vi "velocitymode_rev3_ab.vi"() -> ()   [LabVIEW 2018]
uses:
  <vilib>/rvi/interface/nirviOpenFPGA/nirviOpenFPGA.xnode
  FPGA Bitfiles/WattBalanceRev1_FPGATarget_FPGASPI2_21rs6YSGst0.lvbitx
  <vilib>/rvi/interface/nirviCloseFPGA/nirviCloseFPGA.xnode
  <vilib>/FPGAPlugInAG/Dynamic/niLvFpga_Close_Dynamic.vi
  <vilib>/FPGAPlugInAG/myRIO-1900/niLvFpga_Open_myRIO-1900.vi
  <vilib>/rvi/interface/common/dynamic/niFpgaDynamicAddResources.vi
  <vilib>/Platform/TimedLoop/XDataNode/XDataNode.xnode
  <vilib>/Platform/TimedLoop/XDataNode/nitl_modes.ctl
  <vilib>/Platform/TimedLoop/XDataNode/XDNodeRunTimeDep.lvlib
  <vilib>/Platform/TimedLoop/XDataNode/wakeup.ctl
  <vilib>/Platform/TimedLoop/XDataNode/timing_clust.ctl
panel:
  out "Finished Late? [i-1]":bool
  out "BL":dbl(graph)=0.00030517112470818
  out "x/y":dbl
  out "velocity":dbl(graph)=0.00030517112470818
  out "prev pos":dbl
  in  "emf on/off":bool
  in  "pos on/off":bool
  out "Smooth EMF":dbl(graph)
  out "Smooth position":dbl(graph)=0.00030517112470818
  in  "no. moving avg.":i32=5
  in  "CH1":bool[](array[boolean])=[FALSE, FALSE, TRUE, FALSE, FALSE, TRUE, FALSE, FALSE, FALSE, FALSE, FALSE, FALSE, FALSE, FALSE, FALSE, FALSE]
  in  "CH2":bool[](array[boolean])=[FALSE, FALSE, FALSE, FALSE, FALSE, TRUE, FALSE, FALSE, FALSE, FALSE, FALSE, FALSE, FALSE, FALSE, FALSE, FALSE]
  in  "Color Box 2":u32(colorbox)
  in  "Stop Button":bool
  in  "offset (mV)":dbl
  in  "amplitude (V)":dbl
  in  "frequency (Hz)":dbl
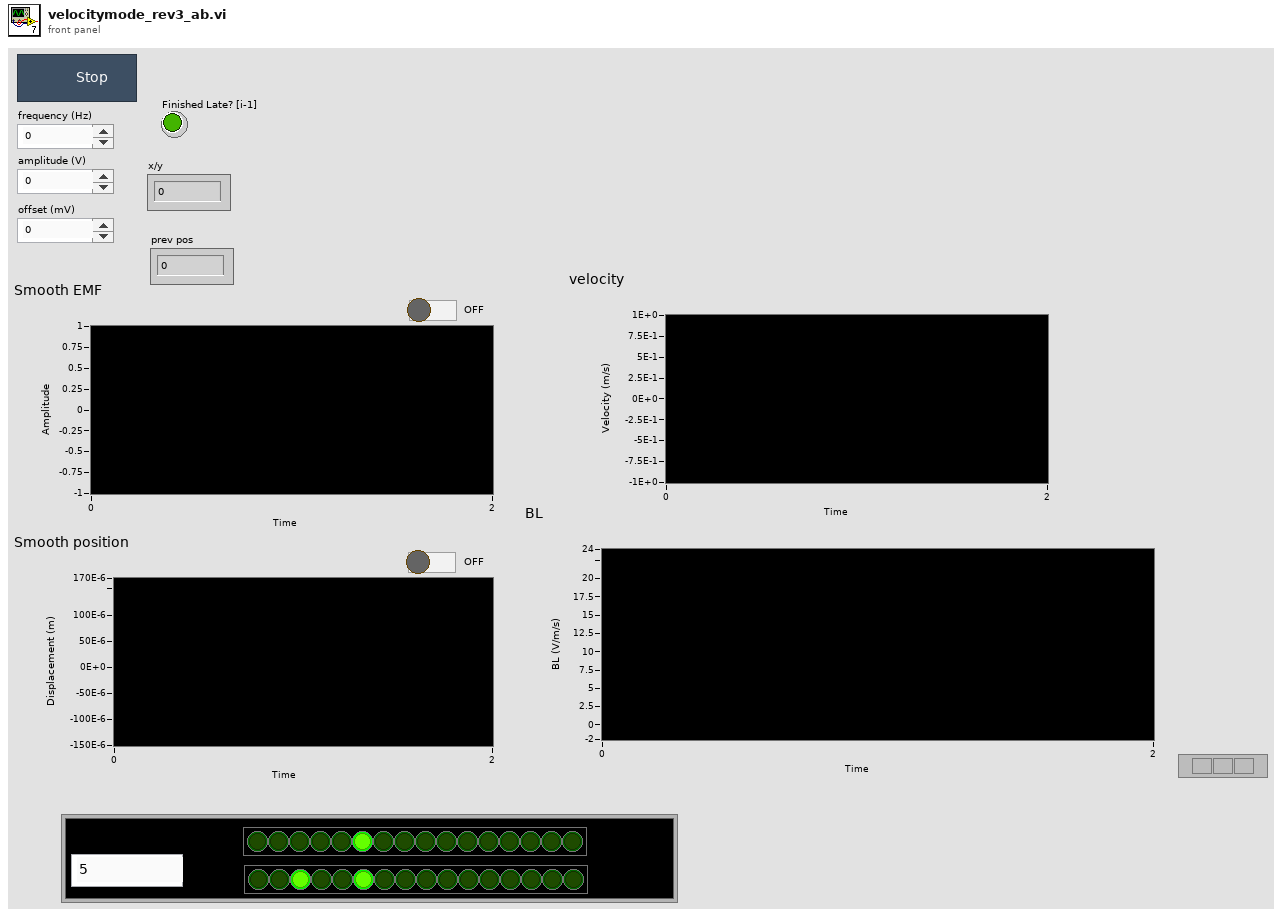
[diagram p1: front panel]
types:
  T1 = typedef "XDNodeRunTimeDep.lvlib/timing_clust.ctl" = cluster{"Expected End [f-1]":u64, "Actual End [f-1]":u64, "Finished Late? [f-1]":bool, "Expected End [i-1]":u64, "Actual End [i-1]":u64, "Finished Late? [i-1]":bool, "Expected Start [i]":u64, "Actual Start [i]":u64, "Expected Start [f]":u64, "Actual Start [f]":u64, "Source Name":string, "Structure Name":string, "Period":i64, "Deadline":i64, "Offset":i64, "Start":i64, "Priority":i32, "Timeout":i32, "Mode":T2, "Wakeup Reason":T3, "Error":errorcluster, "Source Type":string, "Secondary Source Type":string, "Global End Time":u64, "Global Start Time":u64, "Frame Duration":u64, "Iteration Duration":u64, "Assigned CPU":i32, "I/O Scan Engine Mode":u32}
  T2 = typedef "XDNodeRunTimeDep.lvlib/nitl_modes.ctl" = enum32{"No Change", "Process missed periods, maintain original phase", "Discard missed periods, maintain original phase", "Process missed periods, ignore original phase", "Discard missed periods, ignore original phase"}
  T3 = typedef "XDNodeRunTimeDep.lvlib/wakeup.ctl" = enum32{"Normal", "Aborted", "Asynchronous wakeup", "Timing source error", "Timed loop error", "Timeout"}
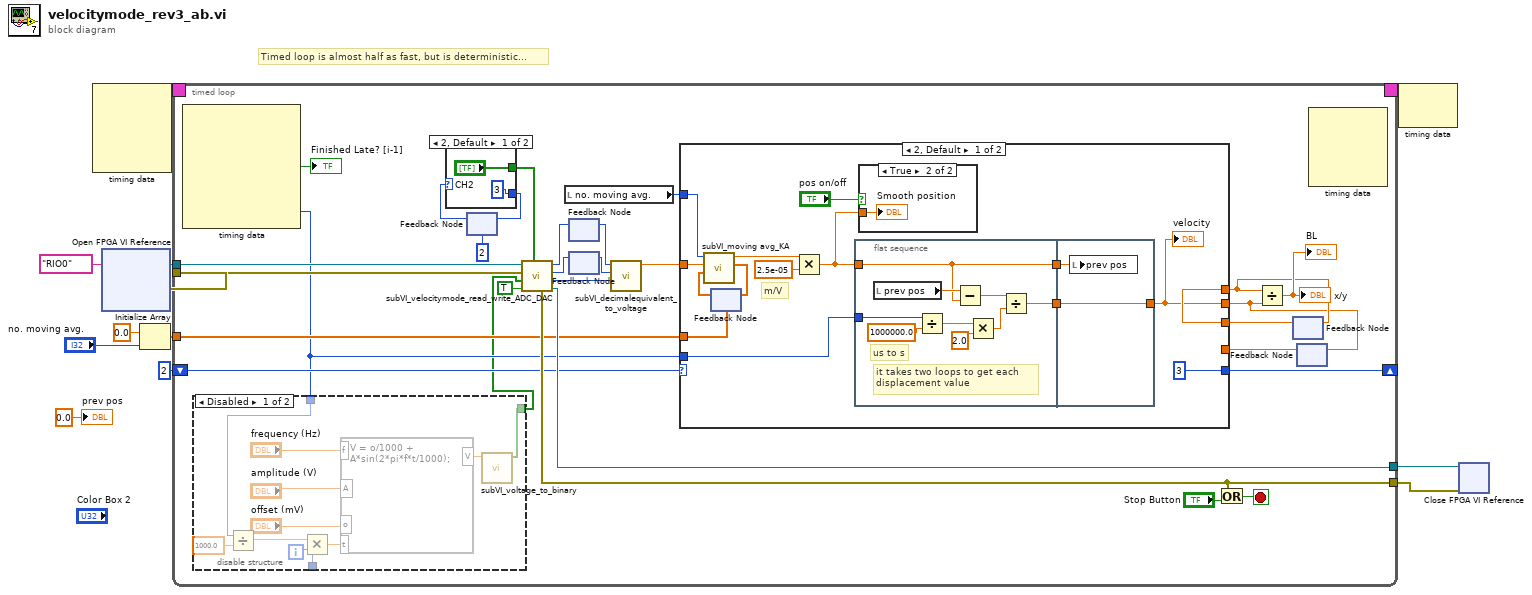
[diagram p0: block diagram]
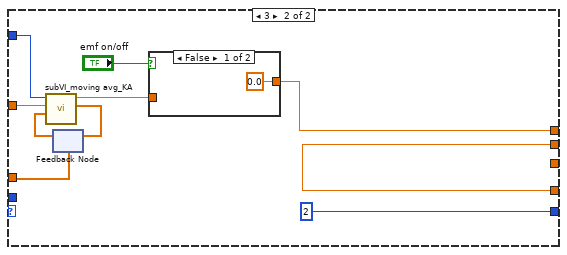
[diagram p4: hidden frame]
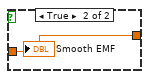
[diagram p5: hidden frame]
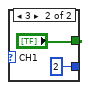
[diagram p6: hidden frame]
diagram:
  # "Timed loop is almost half as fast, but is deterministic..."
  n1 = node-c288() -> (w4:T1)  [unwired: 4 in]
  n2 = xnode "Open FPGA VI Reference"("resource name"=tag "RIO0") -> ("FPGA VI Reference Out"=w12:refnum<k20>, "error out"=w11:errorcluster)  [unwired: 1 in]
  n3 = Initialize Array(0.0 ("element"), "no. moving avg.") -> (w6:dbl[])
  n4 = timed-loop {
    tunnel: w12 -> [w42]
    tunnel: w11 -> [w41]
    tunnel: [w29] -> w10
    tunnel: [w28] -> w9
    tunnel: w6 -> [w25]
    timing: w4 -> [_]
    timing-out: [_] -> w3
    shift-right: [w17] -> _
    shift-left: 2 -> [w18]
    i -> [w16]
    stop <- w31 stop-if-true
    n5 = node-c288() -> (→"Finished Late? [i-1]":bool, w15:i64)  [unwired: 1 in, 5 out]
    n6 = disable-structure shown="Disabled" {
      disable-tunnel: [w48 _] -> w13
      disable-tunnel: w16 -> [w46 _]
      disable-tunnel: w15 -> [w43 _]
      frame Disabled {
        n7 = Divide(x=w43, y=1000.0) -> (x/y=w44:dbl)
        n8 = Multiply(x=w44, y=w46) -> (x*y=w47:dbl)
        n9 = formula code="V = o/1000 + \nA*sin(2*pi*f*t/1000);"("f"="frequency (Hz)", "A"="amplitude (V)", "t"=w47, "o"="offset (mV)") -> ("V"=w49:dbl)
        n10 = call "subVI_voltage_to_binary.vi"("voltage"=w49) -> ("binary"=w48:bool[])  [unwired: 10 in]
      }
      frame Enabled {
      }
    }
    n11 = feedback #1(2) -> (w40:i32)
    n12 = case shown="2, Default" w40 {
      tunnel: ["CH2" "CH1"] -> w38
      tunnel: [3 2] -> w39
      frame 2, Default {
      }
      frame 3 {
      }
    }
    n13 = feedback-in #1(w39) -> ()
    n14 = call "subVI_velocitymode_read_write_ADC_DAC.vi"("CH"=w38, "read only"=TRUE, "DAC1"=w13, "error in"=w41, "FPGA VI Reference In"=w42) -> ("FPGA VI Reference Out"=w29:refnum<k20>, "i"=w34:u32, "GAIN"=w35:i16, "UNI"=w36:i16, "error out"=w28:errorcluster)  [unwired: 2 in]
    n15 = local read "no. moving avg."() -> (w27:i32)
    n16 = feedback-in #2(w36) -> ()
    n17 = feedback #2() -> (w32:i16)  [unwired: 1 in]
    n18 = feedback #3() -> (w33:i16)  [unwired: 1 in]
    n19 = feedback-in #3(w35) -> ()
    n20 = call "subVI_decimalequivalent_to_voltage.vi"("i"=w34, "GAIN"=w33, "UNI"=w32) -> ("V"=w26:dbl)  [unwired: 8 in]
    n21 = Or(x=w28, y="Stop Button") -> (x .or. y?=w31:bool)
    n22 = feedback #4() -> (w24:dbl)  [unwired: 1 in]
    n23 = feedback #5() -> (w23:dbl)  [unwired: 1 in]
    n24 = case shown="2, Default" w18 {
      tunnel: [3 2] -> w17
      tunnel: w27 -> [w70 w89]
      tunnel: w26 -> [w68 w87]
      tunnel: w25 -> [w69 w88]
      tunnel: [w63 w85] -> w21
      tunnel: [w58 w84] -> w20
      tunnel: w24 -> [w63 _]
      tunnel: w23 -> [_ w84]
      tunnel: w15 -> [w57 _]
      frame 2, Default {
        # "m/V"
        n25 = feedback #6(w69) -> (w66:dbl[])
        n26 = call "subVI_moving avg_KA.vi"("input array"=w66, "sample"=w68, "no. moving avg."=w70) -> ("output array"=w67:dbl[], "avg."=w61:dbl)  [unwired: 7 in]
        n27 = feedback-in #6(w67) -> ()
        n28 = Multiply(x=w61, y=2.5e-05) -> (x*y=w60:dbl)
        n29 = flat-sequence {
          tunnel: w57 -> [w73]
          tunnel: w60 -> [w78]
          tunnel: [w78] -> w64
          tunnel: [w72] -> w59
          tunnel: w64 -> [w82]
          tunnel: w59 -> [w81]
          tunnel: [w81] -> w58
          frame #0 {
            # "us to s"
            # "it takes two loops to get each displacement value"
            n30 = local read "prev pos"() -> (w79:dbl)
            n31 = Divide(x=w73, y=1000000.0) -> (x/y=w75:dbl)
            n32 = Subtract(x=w79, y=w78) -> (x-y=w80:dbl)
            n33 = Multiply(x=w75, y=2.0 ("x")) -> (x*y=w74:dbl)
            n34 = Divide(x=w80, y=w74) -> (x/y=w72:dbl)
          }
          frame #1 {
            n35 = local write "prev pos"(w82) -> ()
          }
        }
        n36 = case shown="True" "pos on/off" {
          tunnel: w60 -> [_ w83]
          frame False {
          }
          frame True {
            "Smooth position" <- w83
          }
        }
        "velocity" <- w58
      }
      frame 3 {
        n37 = feedback #7(w88) -> (w92:dbl[])
        n38 = call "subVI_moving avg_KA.vi"("input array"=w92, "sample"=w87, "no. moving avg."=w89) -> ("output array"=w91:dbl[], "avg."=w90:dbl)  [unwired: 7 in]
        n39 = feedback-in #7(w91) -> ()
        n40 = case shown="False" "emf on/off" {
          tunnel: w90 -> [_ w95]
          tunnel: [0.0 ("avg.") w95] -> w85
          frame False {
          }
          frame True {
            "Smooth EMF" <- w95
          }
        }
      }
    }
    n41 = Divide(x=w21, y=w20) -> (x/y=→"x/y" →"BL":dbl)
    n42 = feedback-in #4(w21) -> ()
    n43 = feedback-in #5(w20) -> ()
    n44 = node-c288() -> ()  [unwired: 4 in, 1 out]
  }
  n45 = node-c288(w3) -> ()  [unwired: 1 out]
  n46 = xnode "Close FPGA VI Reference"("FPGA VI Reference In"=w10, "error in"=w9) -> ()  [unwired: 1 out]
  "prev pos" <- 0.0
